vi "03 Python Node.vi"() -> ()   [LabVIEW 2019]
panel:
  out "Gauge":dbl(knob) scale=0.0..10.0
  in  "Slide":dbl(slide)=5.204081632653061 scale=0.0..10.0
  # "Hit the Run arrow and see the Gauge change to the value of the Slide\n\nHit Continuous Run and watch the Gauge change as you vary the Slide"
  # "Hit Cmd E to see the diagram (code)"
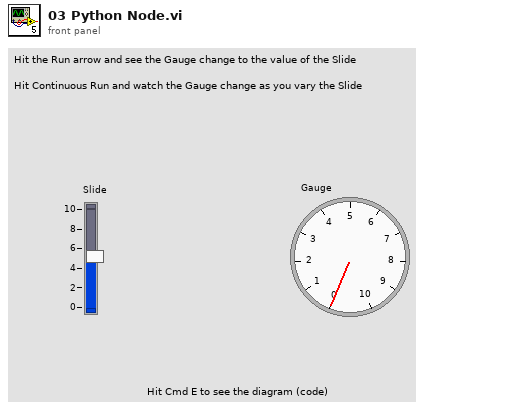
[diagram p1: front panel]
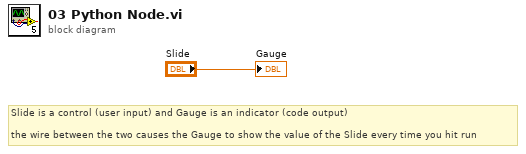
[diagram p0: block diagram]
diagram:
  # "Slide is a control (user input) and Gauge is an indicator (code output)\n\nthe wire between the two causes the Gauge to show the value of the Slide every time you hit run"
  "Gauge" <- "Slide"
